vi "Insert Element at Beginning.vi"(8 "error in (no error)":errorcluster, 10 "element":variant, 11 "Variant in":variant) -> (0 "error out":errorcluster, 3 "Variant out":variant)   [LabVIEW 2017, in "Cluster Manipulation API.lvlib"]
uses:
  Cluster Manipulation API.lvlib
  <vilib>/Utility/Data Type/NI_Data Type.lvlib
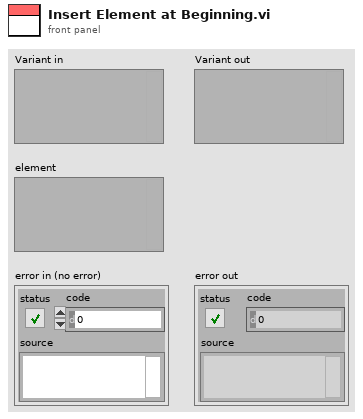
[diagram p1: front panel]
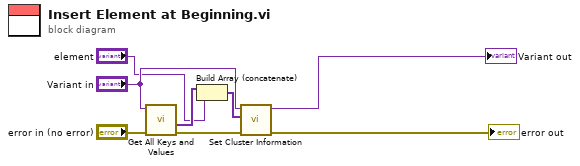
[diagram p0: block diagram]
diagram:
  n1 = call "Get All Keys and Values.vi"("error in"="error in (no error)", "Cluster In"="Variant in") -> ("error out"=w2:errorcluster, "values"=w6:variant[])  [unwired: 6 in, 2 out]
  n2 = Build Array (concatenate)(w6, "element") -> (w1:variant[])
  n3 = call <vilib>:"Set Cluster Information.vi"("error in (no error)"=w2, "Cluster Elements"=w1, "Variant in"="Variant in") -> ("error out"=→"error out":errorcluster, "Variant out"=→"Variant out":variant)  [unwired: 7 in]
